vi "Change All Descriptions.vi"(6 "Prompt?":bool, 9 "new":string, 10 "Path":path, 11 "VI Data in":T1[](array[typedef])) -> (1 "Changed indices":i32[](array[numeric]), 2 "Adjusted All?":bool, 3 "VI Data out":T1[](array[typedef]))   [LabVIEW 2023, in "VI Properties Editor.lvlib"]
uses:
  VI Properties Editor.lvlib
  Cluster Data.ctl
  <vilib>/picture/picture.llb/imagedata.ctl
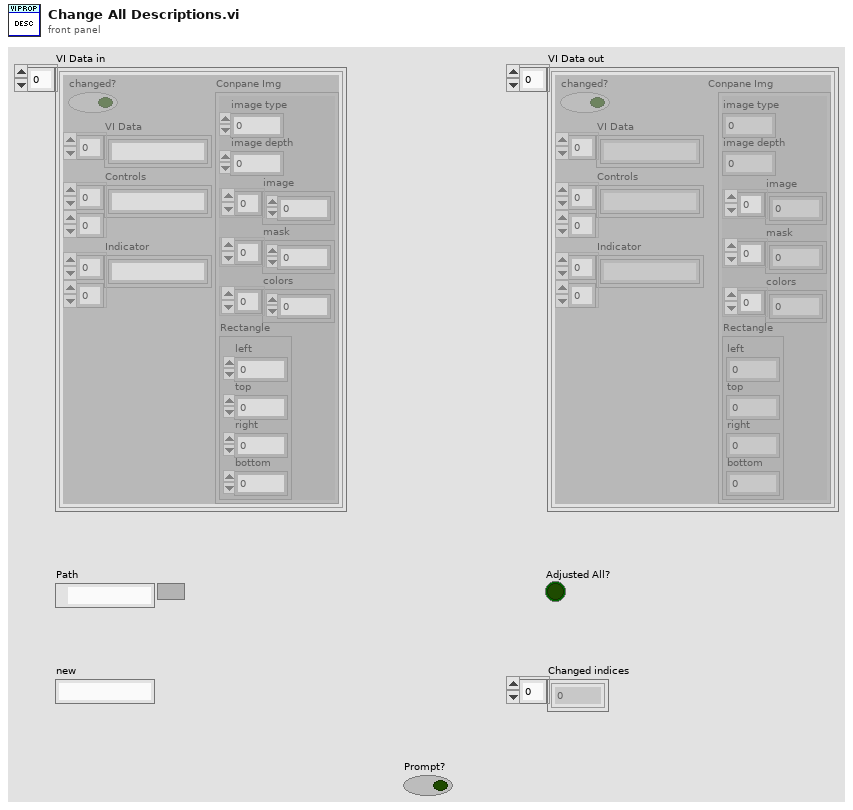
[diagram p1: front panel]
types:
  T1 = typedef "VI Properties Editor.lvlib/Cluster Data.ctl" = cluster{"changed?":bool, "VI Data":string[], "Controls":string[][], "Indicator":string[][], "Conpane Img":T2}
  T2 = typedef "imagedata.ctl" = cluster{"image type":i32, "image depth":i32, "image":u8[], "mask":u8[], "colors":u32[], "Rectangle":cluster{"left":i16, "top":i16, "right":i16, "bottom":i16}}
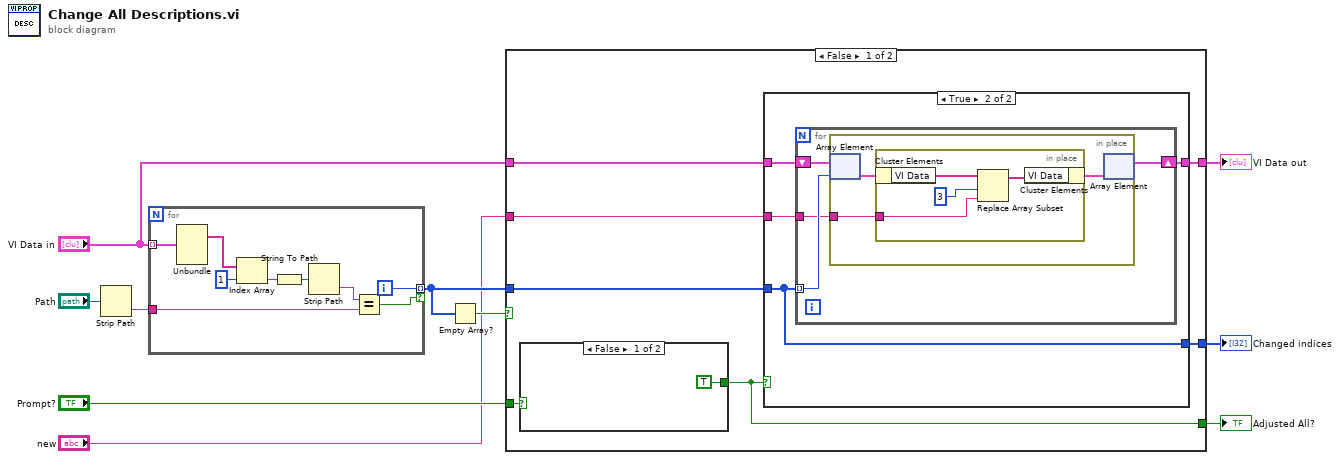
[diagram p0: block diagram]
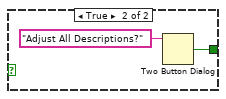
[diagram p2: hidden frame]
diagram:
  n1 = Strip Path(path="Path") -> (name=w9:string)  [unwired: 1 out]
  n2 = for {
    tunnel: "VI Data in" -> [w14] mode=indexing
    tunnel: w9 -> [w16]
    tunnel: [w13] -> w5 mode=indexing if=w12
    i -> [w13]
    n3 = Unbundle(w14) -> ("VI Data"=w11:string[])  [unwired: 4 out]
    n4 = Index Array(array=w11, index=1) -> (element=w18:string)
    n5 = String To Path(string=w18) -> (path=w17:path)
    n6 = Strip Path(path=w17) -> (name=w15:string)  [unwired: 1 out]
    n7 = Equal?(x=w15, y=w16) -> (x = y?=w12:bool)
  }
  n8 = Empty Array?(array=w5) -> (empty?=w7:bool)
  n9 = case shown="False" w7 {
    tunnel: "VI Data in" -> [w25 w46]
    tunnel: [w24 w46] -> w6
    tunnel: w5 -> [w26 _]
    tunnel: "Prompt?" -> [w23 _]
    tunnel: "new" -> [w20 _]
    tunnel: [w22 _] -> w2
    tunnel: [w21 _] -> w1
    frame False {
      n10 = case shown="False" w23 {
        tunnel: [TRUE ("T button?") w28] -> w21
        frame False {
        }
        frame True {
          n11 = Two Button Dialog(message="Adjust All Descriptions?") -> (T button?=w28:bool)  [unwired: 2 in]
        }
      }
      n12 = case shown="True" w21 {
        tunnel: w26 -> [_ w32]
        tunnel: w25 -> [w30 w34]
        tunnel: [w30 w33] -> w24
        tunnel: [_ w32] -> w22
        tunnel: w20 -> [_ w31]
        frame False {
        }
        frame True {
          n13 = for {
            tunnel: w32 -> [w38] mode=indexing
            shift-right: [w37] -> w33
            shift-left: w34 -> [w36]
            tunnel: w31 -> [w35]
            n14 = in-place {
              in-place-border: w35 -> [w39]
              n15 = in-place-array #1(w36, w38) -> (w41:T1)
              n16 = in-place {
                in-place-border: w39 -> [w42]
                n17 = in-place-cluster #2(w41) -> ("VI Data"=w45:string[])
                n18 = Replace Array Subset(array=w45, new element=w42, index=3) -> (w44:string[])
                n19 = in-place-cluster #2("VI Data"=w44) -> (w40:T1)
              }
              n20 = in-place-array #1(w40) -> (w37:T1[])  [unwired: 1 out]
            }
          }
        }
      }
    }
    frame True {
    }
  }
  "VI Data out" <- w6
  "Changed indices" <- w2
  "Adjusted All?" <- w1
